vi "timed loop.vi"() -> ()   [LabVIEW 2025]
uses:
  <vilib>/Platform/TimedLoop/XDataNode/timing_clust.ctl
  <vilib>/Platform/TimedLoop/XDataNode/nitl_modes.ctl
  <vilib>/Platform/TimedLoop/XDataNode/wakeup.ctl
  <vilib>/platform/TimedLoop/XDataNode/XDataNode.xnode
  <vilib>/Platform/TimedLoop/XDataNode/XDNodeRunTimeDep.lvlib
panel:
  out "Numeric 2":dbl
  out "Numeric":dbl
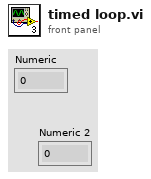
[diagram p1: front panel]
types:
  T1 = typedef "XDNodeRunTimeDep.lvlib/timing_clust.ctl" = cluster{"Expected End [f-1]":u64, "Actual End [f-1]":u64, "Finished Late? [f-1]":bool, "Expected End [i-1]":u64, "Actual End [i-1]":u64, "Finished Late? [i-1]":bool, "Expected Start [i]":u64, "Actual Start [i]":u64, "Expected Start [f]":u64, "Actual Start [f]":u64, "Source Name":string, "Structure Name":string, "Period":i64, "Deadline":i64, "Offset":i64, "Start":i64, "Priority":i32, "Timeout":i32, "Mode":T2, "Wakeup Reason":T3, "Error":errorcluster, "Source Type":string, "Secondary Source Type":string, "Global End Time":u64, "Global Start Time":u64, "Frame Duration":u64, "Iteration Duration":u64, "Assigned CPU":i32, "I/O Scan Engine Mode":u32}
  T2 = typedef "XDNodeRunTimeDep.lvlib/nitl_modes.ctl" = enum32{"No Change", "Process missed periods, maintain original phase", "Discard missed periods, maintain original phase", "Process missed periods, ignore original phase", "Discard missed periods, ignore original phase"}
  T3 = typedef "XDNodeRunTimeDep.lvlib/wakeup.ctl" = enum32{"Normal", "Aborted", "Asynchronous wakeup", "Timing source error", "Timed loop error", "Timeout"}
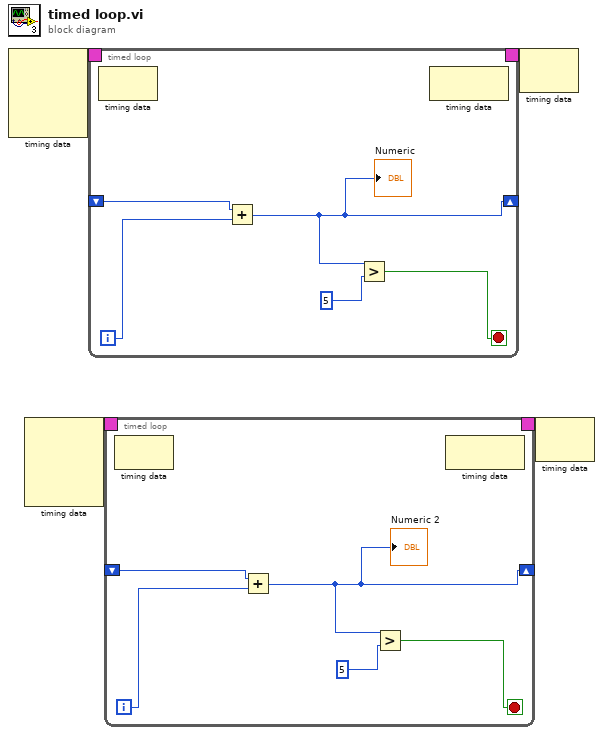
[diagram p0: block diagram]
diagram:
  n1 = node-c288() -> (w4:T1)  [unwired: 4 in]
  n2 = node-c288() -> (w2:T1)  [unwired: 4 in]
  n3 = timed-loop {
    timing: w4 -> [_]
    timing-out: [_] -> w3
    shift-right: [w7] -> _
    shift-left: _ -> [w8]
    i -> [w9]
    stop <- w5 stop-if-true
    n4 = node-c288() -> ()  [unwired: 1 in, 1 out]
    n5 = Add(x=w8, y=w9) -> (x+y=w7:i32)
    "Numeric" <- w7
    n6 = Greater?(x=w7, y=5) -> (0:w5:bool)
    n7 = node-c288() -> ()  [unwired: 1 in, 1 out]
  }
  n8 = timed-loop {
    timing: w2 -> [_]
    timing-out: [_] -> w1
    shift-right: [w14] -> _
    shift-left: _ -> [w15]
    i -> [w16]
    stop <- w12 stop-if-true
    n9 = node-c288() -> ()  [unwired: 1 in, 1 out]
    n10 = Add(x=w15, y=w16) -> (x+y=w14:i32)
    "Numeric 2" <- w14
    n11 = Greater?(x=w14, y=5) -> (0:w12:bool)
    n12 = node-c288() -> ()  [unwired: 1 in, 1 out]
  }
  n13 = node-c288(w3) -> ()  [unwired: 1 out]
  n14 = node-c288(w1) -> ()  [unwired: 1 out]
